vi "Change Modes VBUS.vi"(8 "PhoenixMotorControlDevRef 4":T1={"DeviceStatus"={"status"=FALSE, "code"=0, "source"=""}, "Type"=enum."PWM", "PWM"={"PWM Channel"=enum."PWM 1", "DeadBand"={"Name"="", "maxPositivePwm"=0, "minPositivePwm"=0, "centerPwm"=0, "maxNegativePwm"=0, "minNegativePwm"=0, "angularRange"=0}}, "CAN"={"Device Number"=0, "SetOutput VI Ref"=variant(enum8{"Percent VBus", "Current", "Speed", "Position", "Voltage"} enum."Percent VBus"), "GetOutput VI Ref"=variant(refnum<k1> refnum), "Enable VI Ref"=variant(dbl 12.0), "Disable VI Ref"=variant(enum8{"Percent VBus", "Speed", "Position", "Slave", "Unchanged / Invalid", "Voltage Compensation", "Current", "Motion Profile"} enum."Percent VBus"), "Data"=variant}, "Invert"=FALSE, "DIO PWM"={"PWM \"Enable\" Channel"=enum."Invalid", "DIOChannel"=enum."Invalid", "PWM Rate"=0.0}}, 9 "PhoenixMotorControlDevRef 3":T1={"DeviceStatus"={"status"=FALSE, "code"=0, "source"=""}, "Type"=enum."PWM", "PWM"={"PWM Channel"=enum."PWM 1", "DeadBand"={"Name"="", "maxPositivePwm"=0, "minPositivePwm"=0, "centerPwm"=0, "maxNegativePwm"=0, "minNegativePwm"=0, "angularRange"=0}}, "CAN"={"Device Number"=0, "SetOutput VI Ref"=variant(enum8{"Percent VBus", "Current", "Speed", "Position", "Voltage"} enum."Percent VBus"), "GetOutput VI Ref"=variant(refnum<k1> refnum), "Enable VI Ref"=variant(dbl 12.0), "Disable VI Ref"=variant(enum8{"Percent VBus", "Speed", "Position", "Slave", "Unchanged / Invalid", "Voltage Compensation", "Current", "Motion Profile"} enum."Percent VBus"), "Data"=variant}, "Invert"=FALSE, "DIO PWM"={"PWM \"Enable\" Channel"=enum."Invalid", "DIOChannel"=enum."Invalid", "PWM Rate"=0.0}}, 10 "PhoenixMotorControlDevRef 2":T1={"DeviceStatus"={"status"=FALSE, "code"=0, "source"=""}, "Type"=enum."PWM", "PWM"={"PWM Channel"=enum."PWM 1", "DeadBand"={"Name"="", "maxPositivePwm"=0, "minPositivePwm"=0, "centerPwm"=0, "maxNegativePwm"=0, "minNegativePwm"=0, "angularRange"=0}}, "CAN"={"Device Number"=0, "SetOutput VI Ref"=variant(enum8{"Percent VBus", "Current", "Speed", "Position", "Voltage"} enum."Percent VBus"), "GetOutput VI Ref"=variant(refnum<k1> refnum), "Enable VI Ref"=variant(dbl 12.0), "Disable VI Ref"=variant(enum8{"Percent VBus", "Speed", "Position", "Slave", "Unchanged / Invalid", "Voltage Compensation", "Current", "Motion Profile"} enum."Percent VBus"), "Data"=variant}, "Invert"=FALSE, "DIO PWM"={"PWM \"Enable\" Channel"=enum."Invalid", "DIOChannel"=enum."Invalid", "PWM Rate"=0.0}}, 11 "PhoenixMotorControlDevRef":T1={"DeviceStatus"={"status"=FALSE, "code"=0, "source"=""}, "Type"=enum."PWM", "PWM"={"PWM Channel"=enum."PWM 1", "DeadBand"={"Name"="", "maxPositivePwm"=0, "minPositivePwm"=0, "centerPwm"=0, "maxNegativePwm"=0, "minNegativePwm"=0, "angularRange"=0}}, "CAN"={"Device Number"=0, "SetOutput VI Ref"=variant(enum8{"Percent VBus", "Current", "Speed", "Position", "Voltage"} enum."Percent VBus"), "GetOutput VI Ref"=variant(refnum<k1> refnum), "Enable VI Ref"=variant(dbl 12.0), "Disable VI Ref"=variant(enum8{"Percent VBus", "Speed", "Position", "Slave", "Unchanged / Invalid", "Voltage Compensation", "Current", "Motion Profile"} enum."Percent VBus"), "Data"=variant}, "Invert"=FALSE, "DIO PWM"={"PWM \"Enable\" Channel"=enum."Invalid", "DIOChannel"=enum."Invalid", "PWM Rate"=0.0}}) -> ()   [LabVIEW 2018]
uses:
  <vilib>/Rock Robotics/WPI/MotorControl/WPI_MotorControlDeviceRef.ctl
  <vilib>/Rock Robotics/WPI/MotorControl/WPI_MotorControlType.ctl
  <vilib>/Rock Robotics/SystemInterfaces/DIO/FPGA_DIOPWMChannel.ctl
  <vilib>/Rock Robotics/WPI/PWM/WPI_PWMDeadband.ctl
  <vilib>/Rock Robotics/SystemInterfaces/DIO/FPGA_DIOChannel.ctl
  <vilib>/Rock Robotics/WPI/ThirdParty/Phoenix-LabVIEW/Motor Controller/Controls/CTRE_Phoenix_MotorControl_ControlMode.ctl
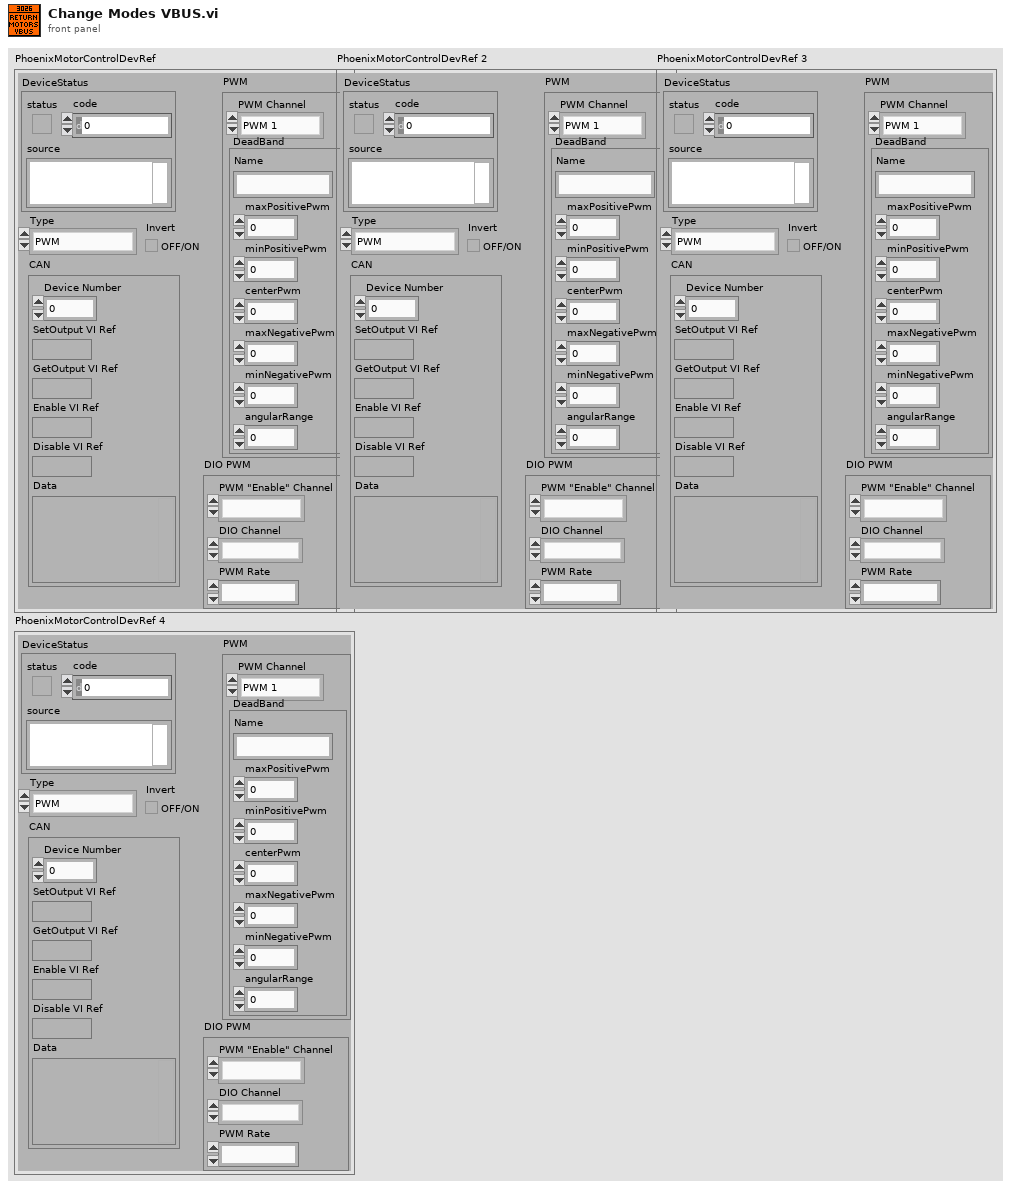
[diagram p1: front panel]
types:
  T1 = typedef "WPI_MotorControlDeviceRef.ctl" = cluster{"DeviceStatus":errorcluster, "Type":T2, "PWM":cluster{"PWM Channel":T3, "DeadBand":T4}, "CAN":cluster{"Device Number":u8, "SetOutput VI Ref":variant, "GetOutput VI Ref":variant, "Enable VI Ref":variant, "Disable VI Ref":variant, "Data":variant}, "Invert":bool, "DIO PWM":cluster{"PWM \"Enable\" Channel":T3, "DIOChannel":T5, "PWM Rate":dbl}}
  T2 = typedef "WPI_MotorControlType.ctl" = enum16{"PWM", "CAN", "DIO PWM"}
  T3 = typedef "FPGA_DIOPWMChannel.ctl" = enum8{"PWM 0", "PWM 1", "PWM 2", "PWM 3", "PWM 4", "PWM 5", "PWM 6", "PWM 7", "PWM 8", "PWM 9", "PWM MXP 0", "PWM MXP 1", "PWM MXP 2", "PWM MXP 3", "PWM MXP 4", "PWM MXP 5", "PWM MXP 6", "PWM MXP 7", "PWM MXP 8", "PWM MXP 9", "Invalid"}
  T4 = typedef "WPI_PWMDeadband.ctl" = cluster{"Name":string, "maxPositivePwm":i32, "minPositivePwm":i32, "centerPwm":i32, "maxNegativePwm":i32, "minNegativePwm":i32, "angularRange":u16}
  T5 = typedef "FPGA_DIOChannel.ctl" = enum8{"DIO 0", "DIO 1", "DIO 2", "DIO 3", "DIO 4", "DIO 5", "DIO 6", "DIO 7", "DIO 8", "DIO 9", "DIO MXP 0", "DIO MXP 1", "DIO MXP 2", "DIO MXP 3", "DIO MXP 4", "DIO MXP 5", "DIO MXP 6", "DIO MXP 7", "DIO MXP 8", "DIO MXP 9", "DIO MXP 10", "DIO MXP 11", "DIO MXP 12", "DIO MXP 13", "DIO MXP 14", "DIO MXP 15", "SPI Port CS1", "SPI Port CS2", "SPI Port CS3", "SPI Port MISO", "SPI Port MOSI", "Invalid"}
  T6 = typedef "CTRE_Phoenix_MotorControl_ControlMode.ctl" = u16
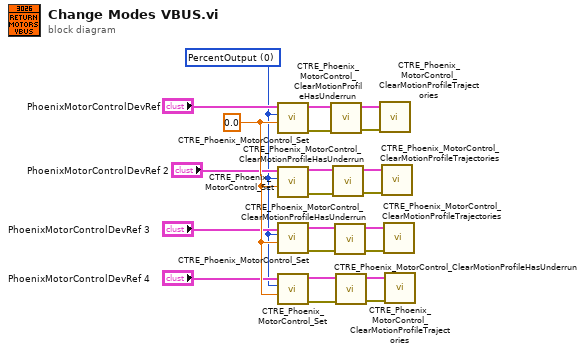
[diagram p0: block diagram]
diagram:
  w17 = T6 0 items=["PercentOutput"=0, "Position"=1, "Velocity"=2, "Follower"=5, "MotionProfile"=6, "MotionMagic"=7, "MotionMagicArc"=8, "TimedPercentOutput"=9, "Disabled"=15] ("Control Mode")
  w22 = 0.0 ("Output")
  n1 = call <vilib>:"CTRE_Phoenix_MotorControl_Set.vi"("Output"=w22, "Control Mode"=w17, "PhoenixMotorControlDevRef"="PhoenixMotorControlDevRef") -> ("error out"=w13:errorcluster, "PhoenixMotorControlDevRef"=w14:T1)  [unwired: 7 in]
  n2 = call <vilib>:"CTRE_Phoenix_MotorControl_Set.vi"("Output"=w22, "Control Mode"=w17, "PhoenixMotorControlDevRef"="PhoenixMotorControlDevRef 2") -> ("error out"=w9:errorcluster, "PhoenixMotorControlDevRef"=w10:T1)  [unwired: 7 in]
  n3 = call <vilib>:"CTRE_Phoenix_MotorControl_Set.vi"("Output"=w22, "Control Mode"=w17, "PhoenixMotorControlDevRef"="PhoenixMotorControlDevRef 3") -> ("error out"=w5:errorcluster, "PhoenixMotorControlDevRef"=w6:T1)  [unwired: 7 in]
  n4 = call <vilib>:"CTRE_Phoenix_MotorControl_Set.vi"("Output"=w22, "Control Mode"=w17, "PhoenixMotorControlDevRef"="PhoenixMotorControlDevRef 4") -> ("error out"=w1:errorcluster, "PhoenixMotorControlDevRef"=w2:T1)  [unwired: 7 in]
  n5 = call <vilib>:"CTRE_Phoenix_MotorControl_ClearMotionProfileHasUnderrun.vi"("error in"=w13, "PhoenixMotorControlDevRef"=w14) -> ("error out"=w15:errorcluster, "PhoenixMotorControlDevRef"=w16:T1)  [unwired: 8 in]
  n6 = call <vilib>:"CTRE_Phoenix_MotorControl_ClearMotionProfileHasUnderrun.vi"("error in"=w9, "PhoenixMotorControlDevRef"=w10) -> ("error out"=w11:errorcluster, "PhoenixMotorControlDevRef"=w12:T1)  [unwired: 8 in]
  n7 = call <vilib>:"CTRE_Phoenix_MotorControl_ClearMotionProfileHasUnderrun.vi"("error in"=w5, "PhoenixMotorControlDevRef"=w6) -> ("error out"=w7:errorcluster, "PhoenixMotorControlDevRef"=w8:T1)  [unwired: 8 in]
  n8 = call <vilib>:"CTRE_Phoenix_MotorControl_ClearMotionProfileHasUnderrun.vi"("error in"=w1, "PhoenixMotorControlDevRef"=w2) -> ("error out"=w3:errorcluster, "PhoenixMotorControlDevRef"=w4:T1)  [unwired: 8 in]
  n9 = call <vilib>:"CTRE_Phoenix_MotorControl_ClearMotionProfileTrajectories.vi"("PhoenixMotorControlDevRef"=w16, "error in"=w15) -> ()  [unwired: 12 in, 2 out]
  n10 = call <vilib>:"CTRE_Phoenix_MotorControl_ClearMotionProfileTrajectories.vi"("PhoenixMotorControlDevRef"=w12, "error in"=w11) -> ()  [unwired: 12 in, 2 out]
  n11 = call <vilib>:"CTRE_Phoenix_MotorControl_ClearMotionProfileTrajectories.vi"("PhoenixMotorControlDevRef"=w8, "error in"=w7) -> ()  [unwired: 12 in, 2 out]
  n12 = call <vilib>:"CTRE_Phoenix_MotorControl_ClearMotionProfileTrajectories.vi"("PhoenixMotorControlDevRef"=w4, "error in"=w3) -> ()  [unwired: 12 in, 2 out]
